vi "Get Click Position.vi"(10 "Coordinates":T1, 11 "Intensity Graph Ref":refnum<vi>) -> (3 "Click Position":cluster{i32, i32})   [LabVIEW 2018]
doc: "Converts click position from screen pixel coordinates to graph coordinates."
uses:
  <vilib>/Utility/miscctls.llb/LVPoint32TypeDef.ctl
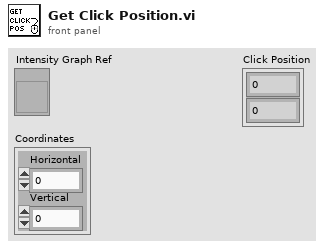
[diagram p1: front panel]
types:
  T1 = typedef "LVPoint32TypeDef.ctl" = cluster{"Horizontal":i32, "Vertical":i32}
  T2 = typedef "LVRectTypeDef.ctl" = cluster{"Left":i16, "Top":i16, "Right":i16, "Bottom":i16}
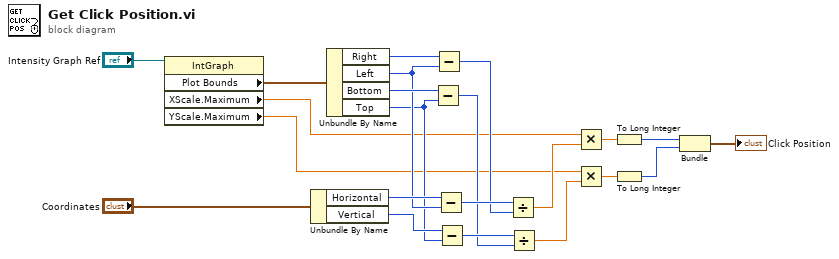
[diagram p0: block diagram]
diagram:
  n1 = property class="IntGraph"(reference="Intensity Graph Ref") -> ("Plot Bounds"=w22:T2, "XScale.Maximum"=w11:dbl, "YScale.Maximum"=w9:dbl)  [unwired: 1 in, 2 out]
  n2 = Unbundle By Name("Coordinates") -> ("Horizontal"=w19:i32, "Vertical"=w17:i32)
  n3 = Unbundle By Name(w22) -> ("Right"=w21:i16, "Left"=w18:i16, "Bottom"=w20:i16, "Top"=w16:i16)
  n4 = Subtract(x=w20, y=w16) -> (x-y=w12:i16)
  n5 = Subtract(x=w21, y=w18) -> (x-y=w13:i16)
  n6 = Subtract(x=w19, y=w18) -> (x-y=w15:i32)
  n7 = Subtract(x=w17, y=w16) -> (x-y=w14:i32)
  n8 = Divide(x=w15, y=w13) -> (x/y=w10:dbl)
  n9 = Divide(x=w14, y=w12) -> (x/y=w8:dbl)
  n10 = Multiply(x=w11, y=w10) -> (x*y=w7:dbl)
  n11 = Multiply(x=w9, y=w8) -> (x*y=w6:dbl)
  n12 = To Long Integer(number=w7) -> (32bit integer=w3:i32)
  n13 = To Long Integer(number=w6) -> (32bit integer=w2:i32)
  n14 = Bundle(w3, w2) -> (→"Click Position":cluster{i32, i32})  [unwired: 1 in]
